vi "Get Path Regex.vi"(8 "error in (no error)":errorcluster, 11 "Test Index in":refnum<class "Test Index.lvclass">) -> (0 "error out":errorcluster, 2 "Path Regex":string, 3 "Test Index out":refnum<class "Test Index.lvclass">)   [LabVIEW 2020, in "Test Index.lvclass"]
uses:
  Test Index.lvclass
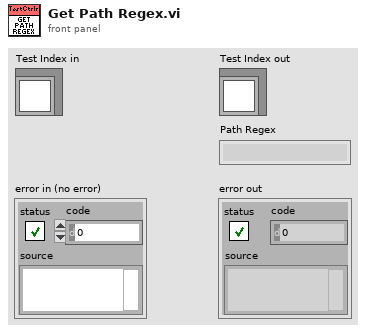
[diagram p1: front panel]
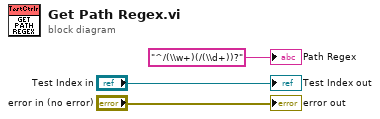
[diagram p0: block diagram]
diagram:
  "error out" <- "error in (no error)"
  "Test Index out" <- "Test Index in"
  "Path Regex" <- "^/(\\w+)(/(\\d+))?" ("Path Regex")
